vi "View.vi"(8 "error out":errorcluster, 11 "2-Axis Stage":refnum<class "2-Axis Stage Async API.lvclass">) -> (0 "error out":errorcluster)   [LabVIEW 2022 SP3, in "Control.lvlib"]
uses:
  Control.lvlib
  Interfaces/2-Axis Stage API/2-Axis Stage Async API.lvclass
panel:
  out "XY Position Graph":cluster{"X":dbl, "Y":dbl}[](graph)
  in  "Abort Motion":bool
  in  "Home Stage":bool
  in  "Move Stage":bool
  in  "Y-Destination":dbl
  in  "X-Destination":dbl
  in  "Clear Error":bool
  out "Y-Speed":dbl
  in  "Set Y-Speed":u16
  in  "Set Y-Acceleration":u16
  out "Y-Current Speed":dbl
  out "Y-Acceleration":dbl
  out "Y-Homed":bool
  out "Y-Moving":bool
  out "Y-Position":dbl
  out "X-Speed":dbl
  in  "Set X-Speed":u16
  in  "Set X-Acceleration":u16
  out "X-Current Speed":dbl
  out "X-Acceleration":dbl
  out "X-Homed":bool
  out "X-Moving":bool
  out "X-Position":dbl
  out "Stage Error":errorcluster
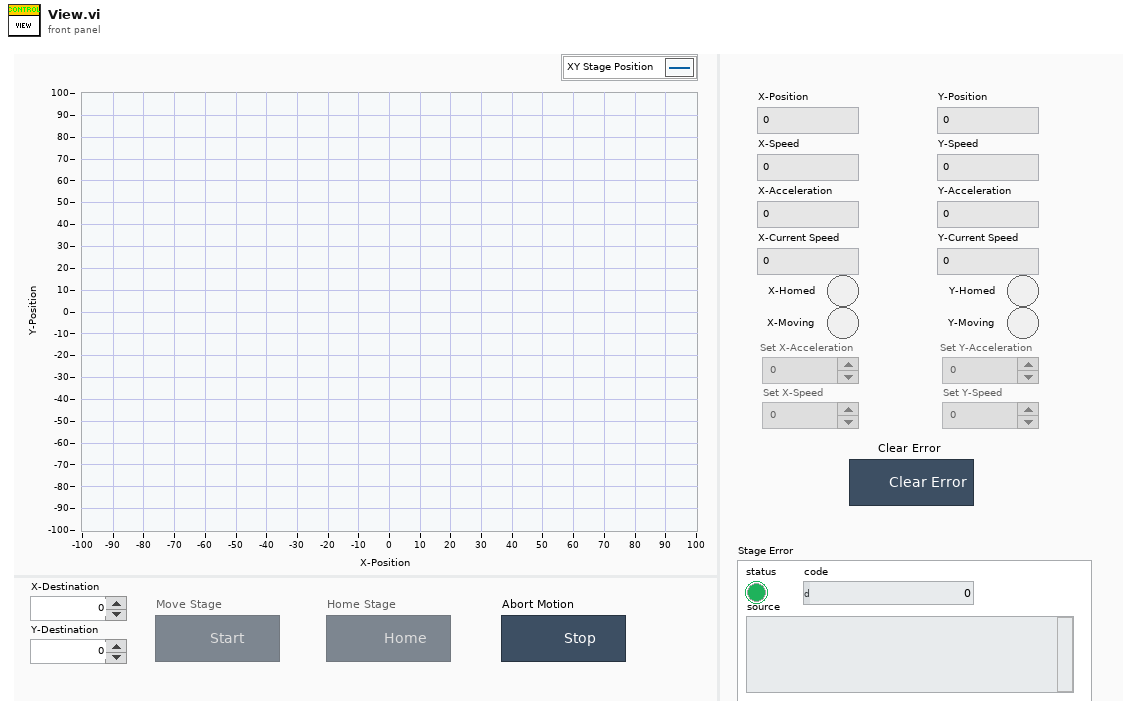
[diagram p1: front panel]
types:
  T1 = enum32{"Invalid", "Standard", "Closed", "Hidden", "Minimized", "Maximized"}
  T2 = enum32{"invalid app kind", "Development System", "Run Time System", "Student Edition", "Embedded LabVIEW", "Evaluation", "Custom"}
  T3 = enum8{"Enabled", "Disabled", "Disabled and Grayed Out"}
  T4 = cluster{"Current Position X":dbl, "Current Position Y":dbl}[]
  T5 = cluster{"Core":cluster{"Current VI Reference":refnum<vi>, "Close Panel on Exit?":bool}, "2-Axis Stage":refnum<class "2-Axis Stage Async API.lvclass">}
  T6 = cluster{"Current VI Reference":refnum<vi>, "Close Panel on Exit?":bool}
  T7 = cluster{"Event Registration Refnum":refnum<event-registration>, "Event Registration Refnum":refnum<event-registration>}
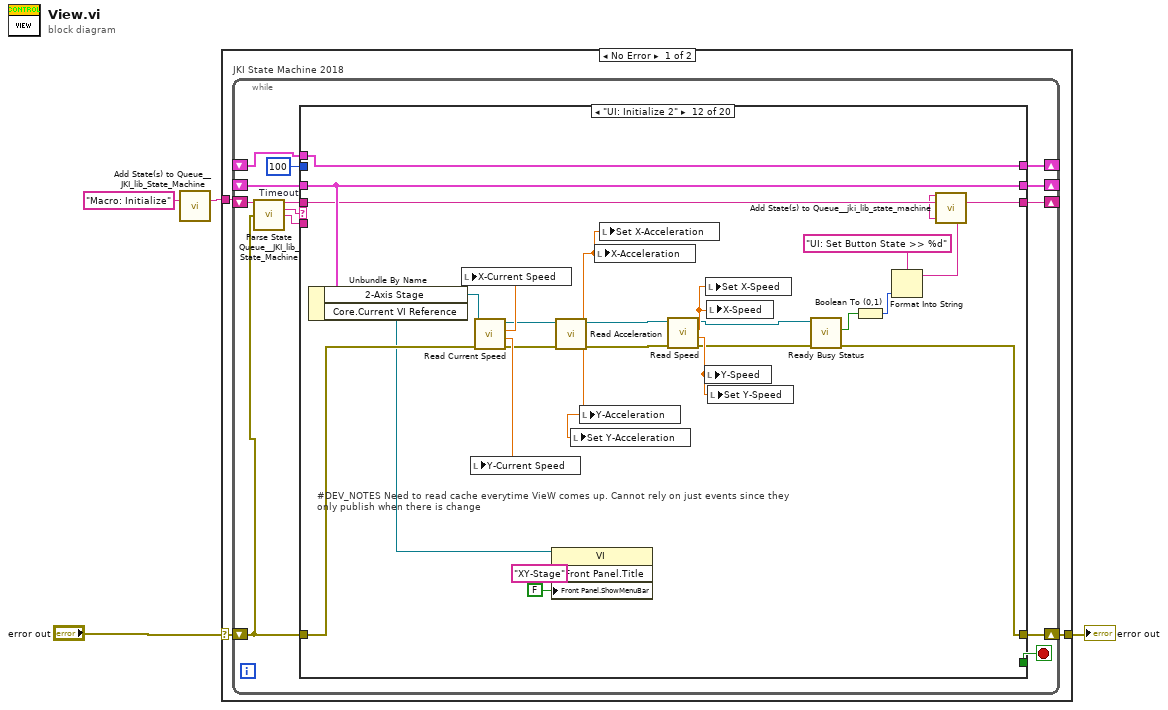
[diagram p0: block diagram]
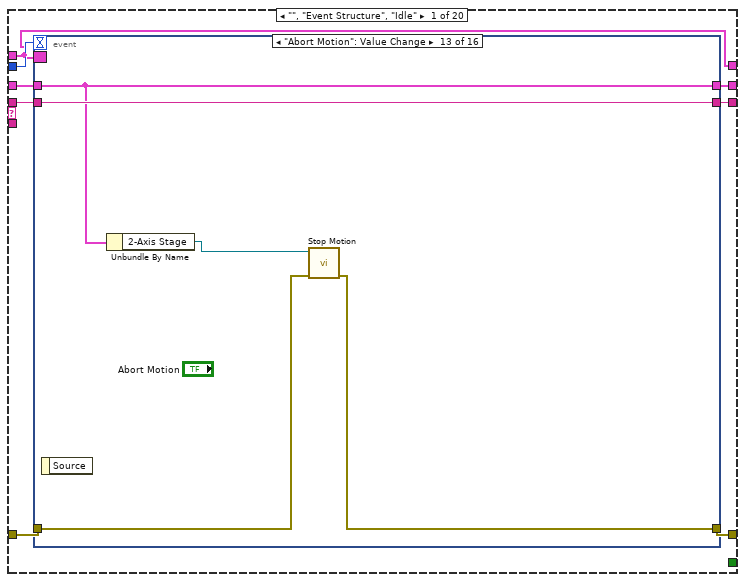
[diagram p2: hidden frame]
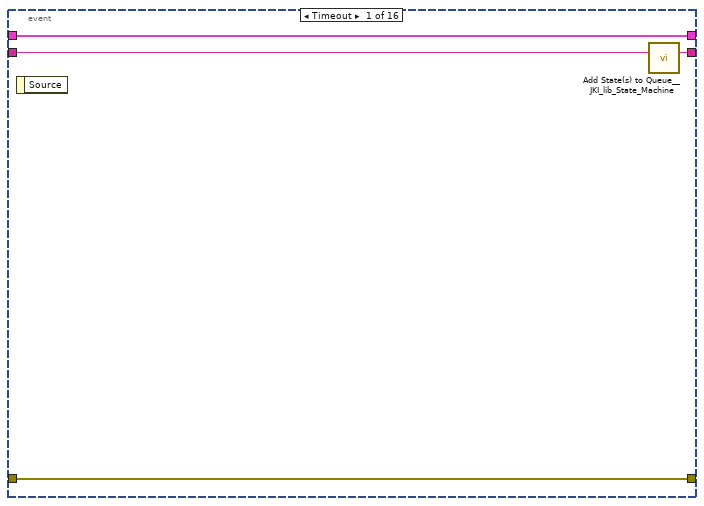
[diagram p3: hidden frame]
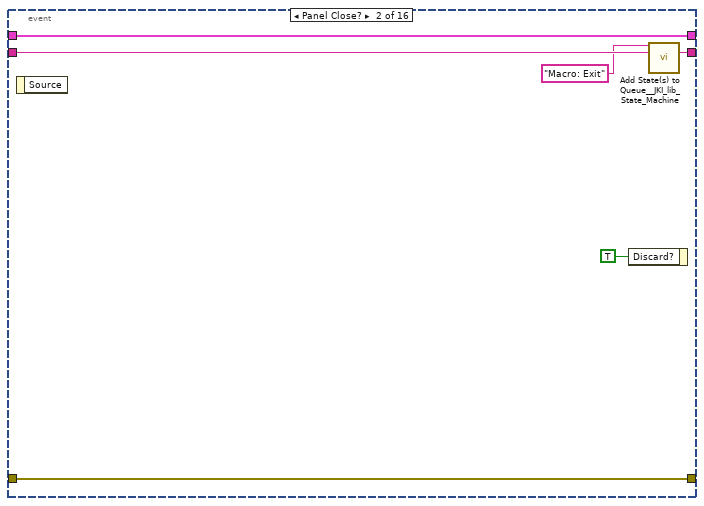
[diagram p4: hidden frame]
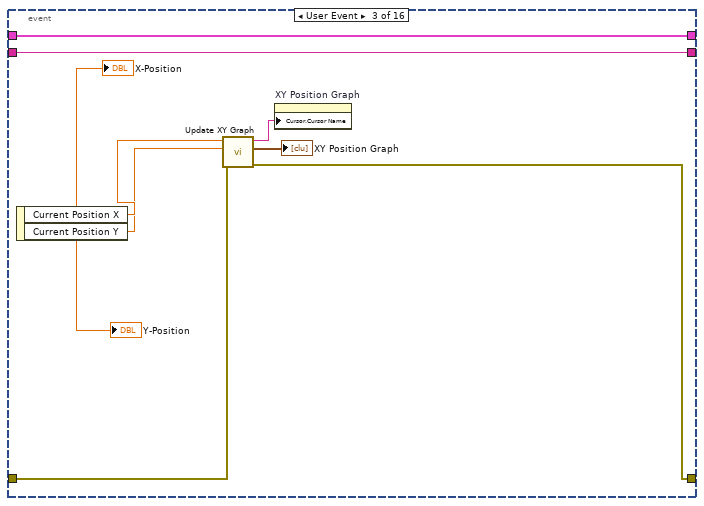
[diagram p5: hidden frame]
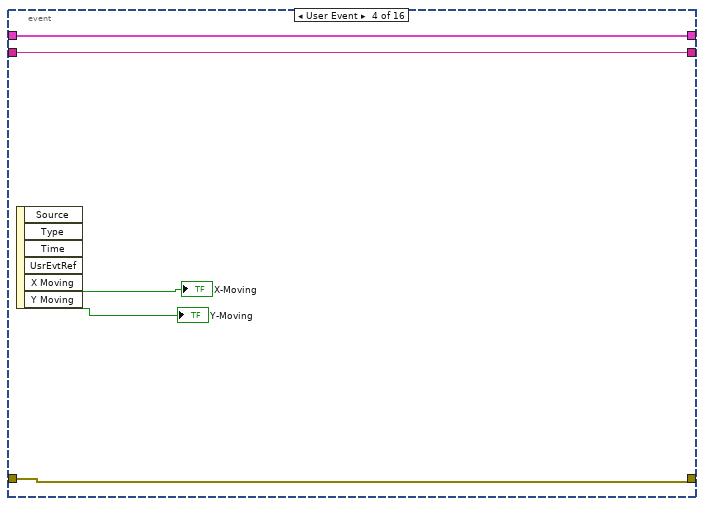
[diagram p6: hidden frame]
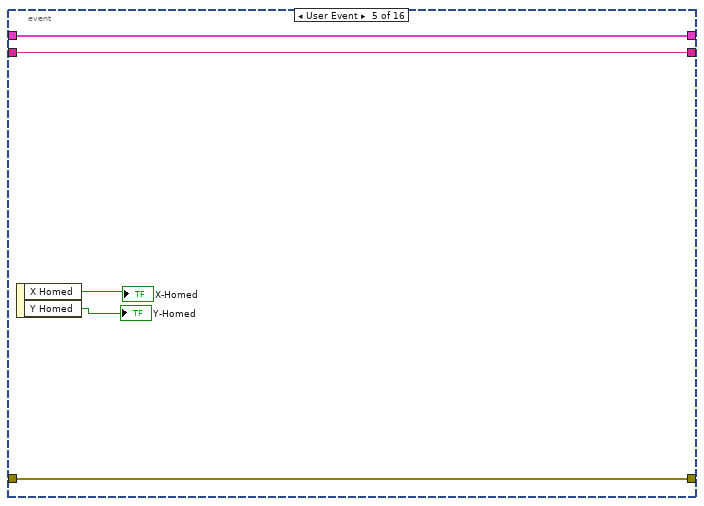
[diagram p7: hidden frame]
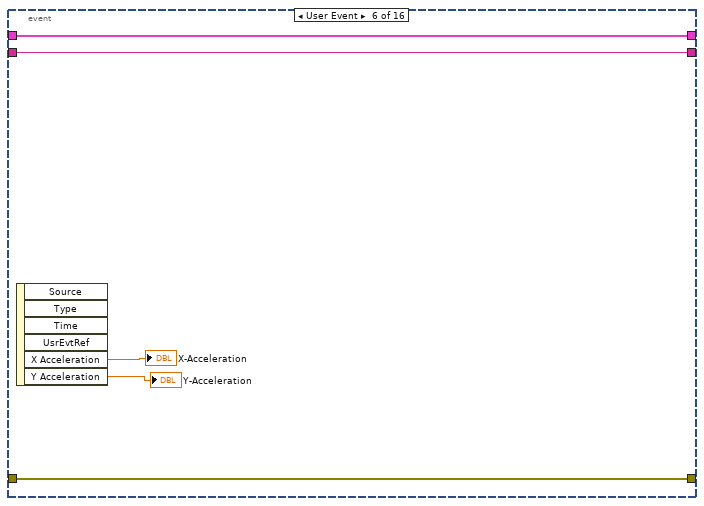
[diagram p8: hidden frame]
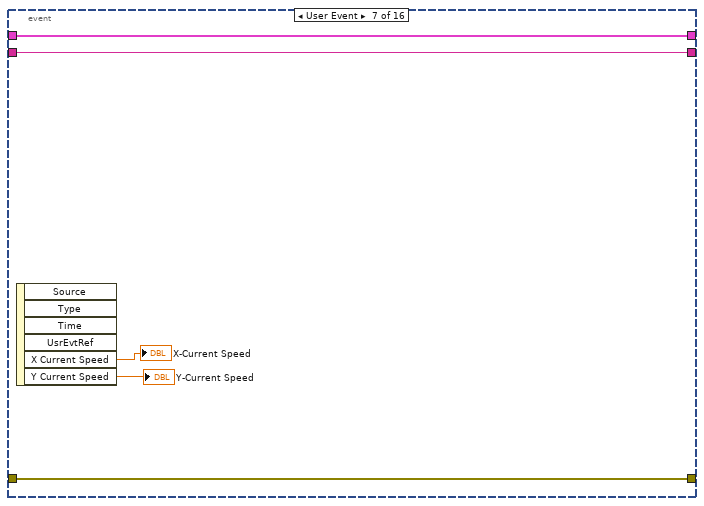
[diagram p9: hidden frame]
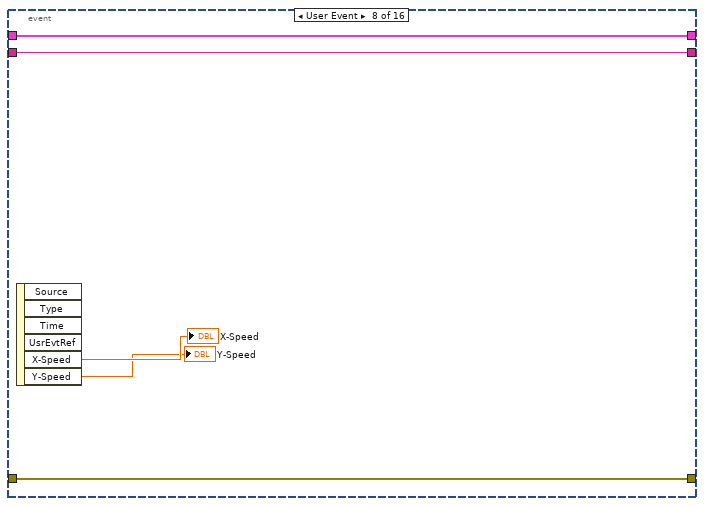
[diagram p10: hidden frame]
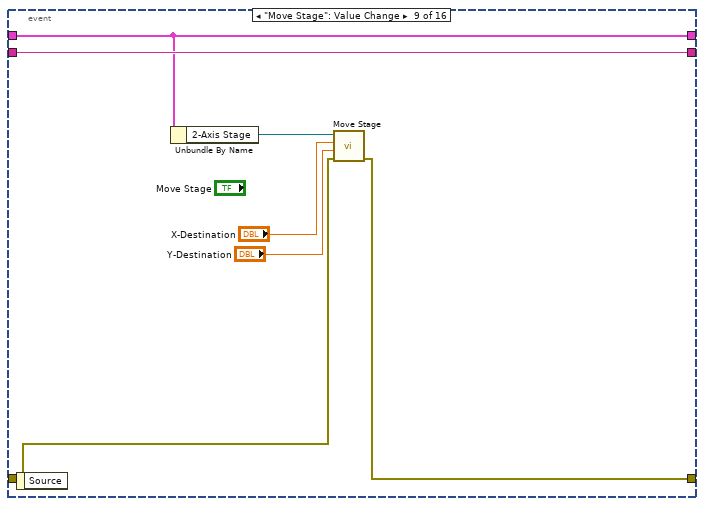
[diagram p11: hidden frame]
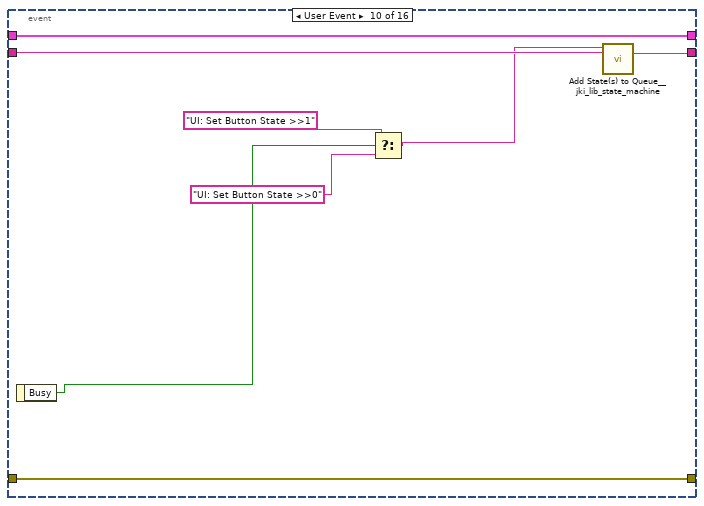
[diagram p12: hidden frame]
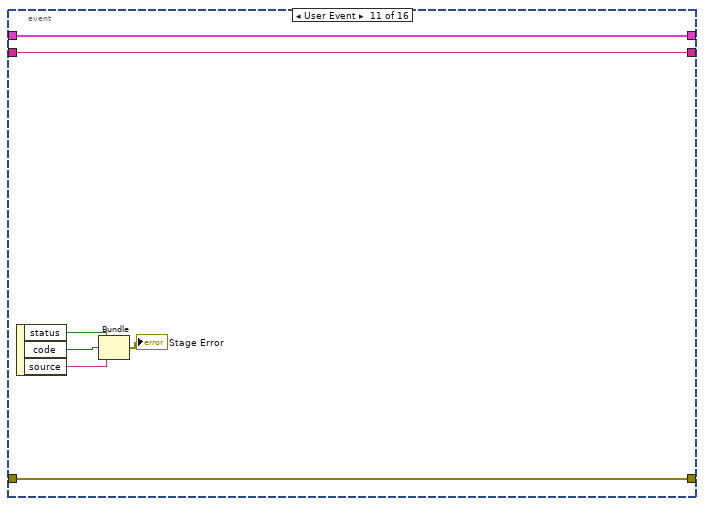
[diagram p13: hidden frame]
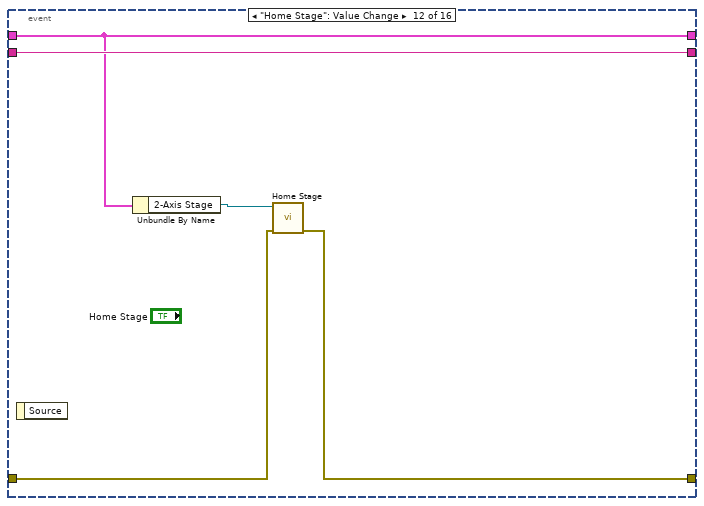
[diagram p14: hidden frame]
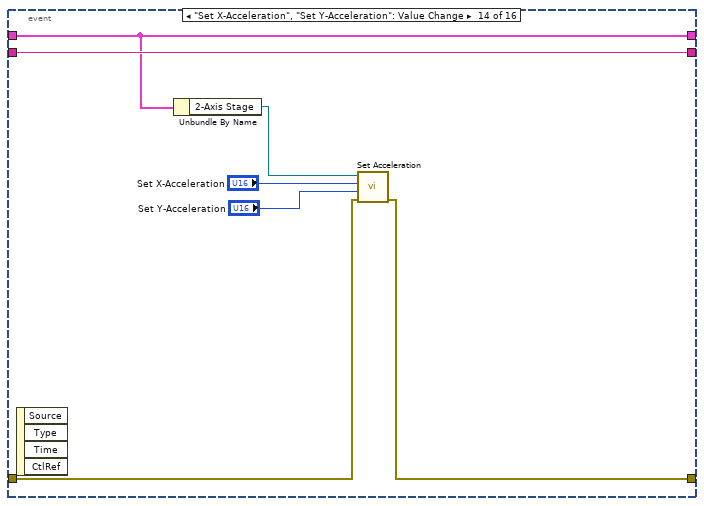
[diagram p15: hidden frame]
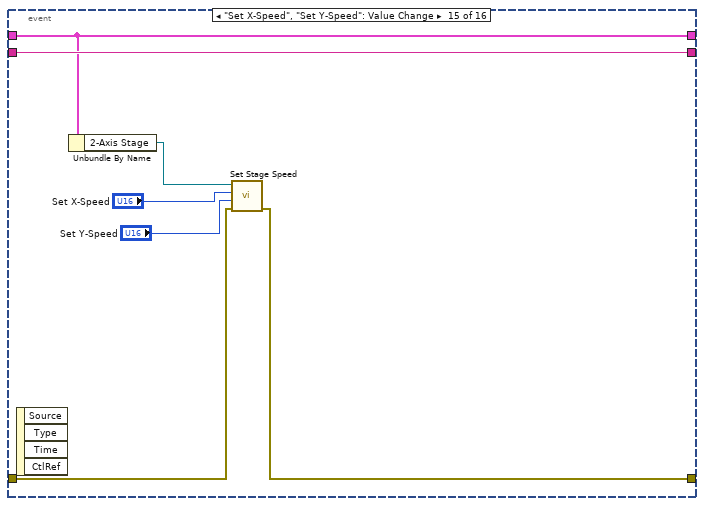
[diagram p16: hidden frame]
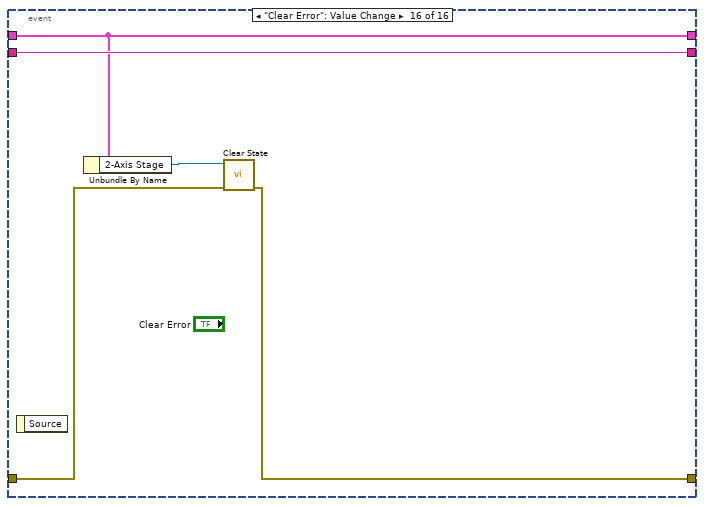
[diagram p17: hidden frame]
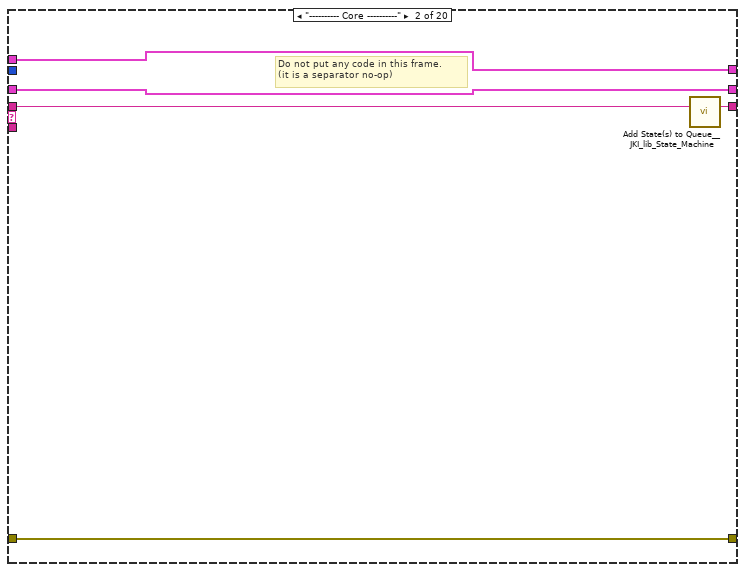
[diagram p18: hidden frame]
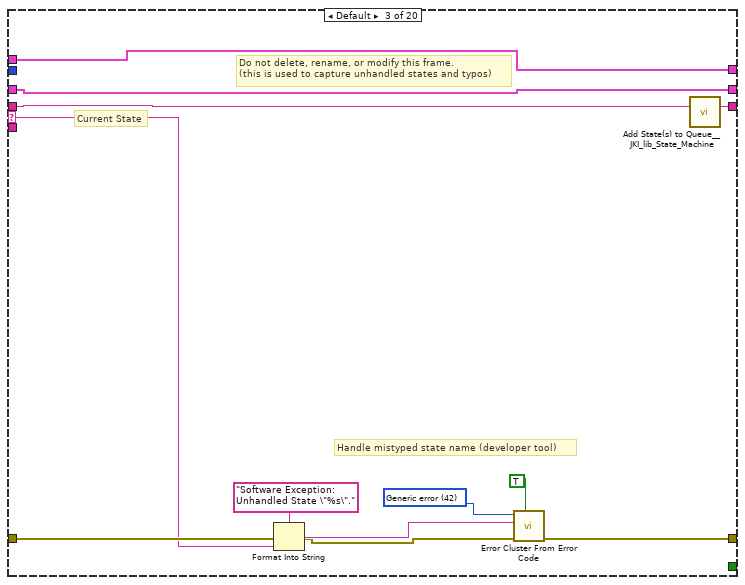
[diagram p19: hidden frame]
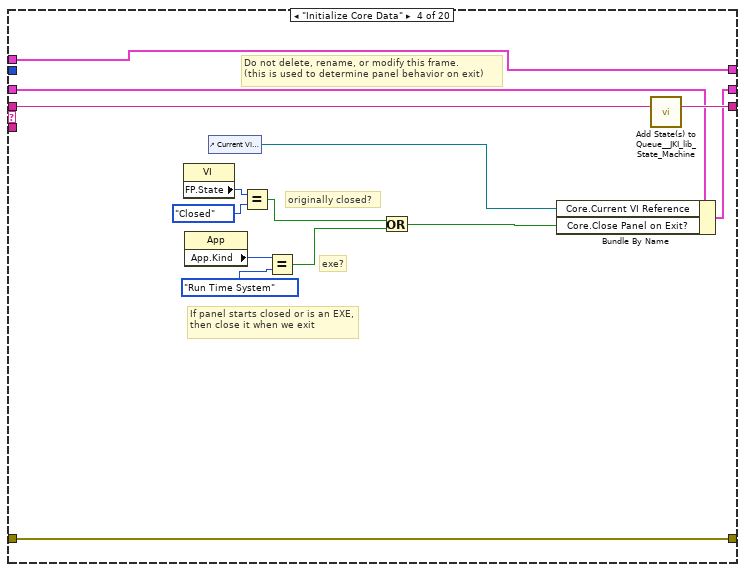
[diagram p20: hidden frame]
diagram:
  n1 = call <vilib>:"Add State(s) to Queue__JKI_lib_State_Machine.vi"("State(s) in (\"\")"="Macro: Initialize") -> ("States Out"=w1:string)  [unwired: 14 in]
  n2 = case shown="No Error" "error out" {
    selector: "error out" -> [w7 _]
    tunnel: [w6 _] -> w3
    tunnel: w1 -> [w5 _]
    frame No Error {
      n3 = while "JKI State Machine 2018" {
        shift-right: [w13] -> _
        shift-left: _ -> [w12]
        shift-right: [w16] -> w6
        shift-left: w7 -> [w10]
        shift-right: [w15] -> _
        shift-left: w5 -> [w17]
        shift-right: [w9] -> _
        shift-left: _ -> [w8]
        stop <- w14 stop-if-true
        w11 = 100  # Timeout
        n4 = call <vilib>:"Parse State Queue__JKI_lib_State_Machine.vi"("State Queue"=w17, "Error In (no error)"=w10) -> ("Remaining States"=w19:string, "Current State"=w20:string, "Arguments"=w18:string)  [unwired: 11 in]
        n5 = case shown="\"UI: Initialize 2\"" w20 {
          selector: w20 -> [_ _ w129 _ _ _ _ _ _ _ _ _ _ _ _ _ _ _ _ _]
          tunnel: w19 -> [w28 w127 w133 w153 w160 w166 w171 w178 w185 w190 w213 w224 w256 w278 w290 w360 w366 w377 w382 w388]
          tunnel: w18 -> [_ _ _ _ _ _ _ _ _ _ _ _ w245 w273 w284 _ _ _ _ _]
          tunnel: w12 -> [w26 w124 w131 w146 w157 w164 w168 _ w180 w187 w210 w228 w247 w276 w286 w357 w363 w374 w379 w387]
          tunnel: [w25 w125 w135 w150 errorcluster {"status"=FALSE, "code"=0, "source"=""} ("error out") w163 w169 w175 w181 w188 w195 w219 w242 w274 w287 w358 w364 w375 w380 w383] -> w16
          tunnel: w10 -> [w24 w125 w134 w150 w154 w163 w169 w175 w182 w188 w202 w226 w241 w275 w288 w358 w364 w375 w380 w384]
          tunnel: [w27 w126 w132 w152 w159 w165 w170 w177 w184 w189 w212 w225 w256 w277 w289 w359 w365 w376 w381 w388] -> w15
          tunnel: [_ _ _ _ _ TRUE _ _ _ _ _ _ _ _ _ _ _ _ _ _] -> w14
          tunnel: [w23 w124 w131 w151 w157 w164 w168 w176 w180 w187 w210 w228 w247 w276 w286 w357 w363 w374 w379 w387] -> w13
          tunnel: w11 -> [w22 _ _ _ _ _ _ _ _ _ _ _ _ _ _ _ _ _ _ _]
          tunnel: [w21 w123 w128 w140 w155 w161 w167 w172 w179 w186 w211 w239 w248 w272 w283 w356 w362 w367 w378 w385] -> w9
          tunnel: w8 -> [w21 w123 w128 w140 w155 w161 w167 w172 w179 w186 w211 w239 w248 w272 w283 w356 w362 w367 w378 _]
          frame "", "Event Structure", "Idle" {
            n6 = event shown="[12] \"Abort Motion\": Value Change" {
              selector: w21 -> [_ _ _ _ _ _ _ _ _ _ _ _ _ _ _ _]
              dyn-events: _ -> [_ _ _ _ _ _ _ _ _ _ _ _ _ _ _ _]
              timeout: w22 -> [_ _ _ _ _ _ _ _ _ _ _ _ _ _ _ _]
              tunnel: w28 -> [w32 w38 w45 w51 w56 w61 w66 w71 w78 w83 w93 w98 w103 w110 w117 w122]
              tunnel: [w31 w37 w45 w51 w56 w61 w66 w71 w78 w84 w93 w98 w103 w110 w117 w122] -> w27
              tunnel: w26 -> [w29 w35 w46 w50 w55 w60 w65 w70 w77 w86 w92 w97 w102 w109 w116 w121]
              tunnel: [w30 w36 w39 w47 w52 w57 w62 w67 w72 w85 w87 w94 w100 w104 w113 w118] -> w25
              tunnel: w24 -> [w30 w36 w40 w47 w52 w57 w62 w67 w73 w85 w87 w95 w99 w105 w114 w119]
              tunnel: [w29 w35 w46 w50 w55 w60 w65 w70 w77 w86 w92 w97 w102 w109 w116 w121] -> w23
              event Timeout {
                n7 = event-data() -> ()  [unwired: 1 in, 1 out]
                n8 = call <vilib>:"Add State(s) to Queue__JKI_lib_State_Machine.vi"("State(s) in (\"\")"=w32) -> ("States Out"=w31:string)  [unwired: 14 in]
              }
              event Panel Close? {
                n9 = event-data() -> ()  [unwired: 1 in, 1 out]
                n10 = event-data("Discard?"=TRUE) -> ()  [unwired: 1 in, 1 out]
                n11 = call <vilib>:"Add State(s) to Queue__JKI_lib_State_Machine.vi"("State(s) in Front (\"\")"="Macro: Exit", "State(s) in (\"\")"=w38) -> ("States Out"=w37:string)  [unwired: 13 in]
              }
              event User Event {
                n12 = event-data() -> ("Current Position X"=w43:dbl, "Current Position Y"=w42:dbl)  [unwired: 1 in]
                "Y-Position" <- w42
                "X-Position" <- w43
                n13 = call "Update XY Graph.vi"("error in (no error)"=w40, "Current Position Y"=w42, "Current Position X"=w43) -> ("error out"=w39:errorcluster, "Array"=→"XY Position Graph":T4, "String"=w41:string)  [unwired: 6 in]
                n14 = property on="XY Position Graph" class="XYGraph (strict)"("Cursor.Cursor Name"=w41) -> ()  [unwired: 2 in, 2 out]
              }
              event User Event {
                n15 = event-data() -> ("X Moving"=→"X-Moving":bool, "Y Moving"=→"Y-Moving":bool)  [unwired: 1 in, 4 out]
              }
              event User Event {
                n16 = event-data() -> ("X Homed"=→"X-Homed":bool, "Y Homed"=→"Y-Homed":bool)  [unwired: 1 in]
              }
              event User Event {
                n17 = event-data() -> ("X Acceleration"=→"X-Acceleration":dbl, "Y Acceleration"=→"Y-Acceleration":dbl)  [unwired: 1 in, 4 out]
              }
              event User Event {
                n18 = event-data() -> ("X Current Speed"=→"X-Current Speed":dbl, "Y Current Speed"=→"Y-Current Speed":dbl)  [unwired: 1 in, 4 out]
              }
              event User Event {
                n19 = event-data() -> ("X-Speed"=→"X-Speed":dbl, "Y-Speed"=→"Y-Speed":dbl)  [unwired: 1 in, 4 out]
              }
              event "Move Stage": Value Change {
                n20 = event-data() -> ()  [unwired: 1 in, 1 out]
                n21 = Unbundle By Name(w77) -> ("2-Axis Stage"=w76:refnum<class "2-Axis Stage Async API.lvclass">)
                n22 = call-dynamic "Move Stage.vi"("error in (no error)"=w73, "Y Axis"="Y-Destination", "X Axis"="X-Destination", "2-Axis Stage in"=w76) -> ("error out"=w72:errorcluster)  [unwired: 6 in, 1 out]
              }
              event User Event {
                n23 = event-data() -> ("Busy"=w82:bool)  [unwired: 1 in]
                n24 = Select(t="UI: Set Button State >>1", s=w82, f="UI: Set Button State >>0") -> (s? t:f=w79:string)
                n25 = call <vilib>:"Add State(s) to Queue__jki_lib_state_machine.vi"("State(s) in Front (\"\")"=w79, "State(s) in (\"\")"=w83) -> ("States Out"=w84:string)  [unwired: 13 in]
              }
              event User Event {
                n26 = event-data() -> ("status"=w91:bool, "code"=w90:i32, "source"=w89:string)  [unwired: 1 in]
                n27 = Bundle("status"=w91, "code"=w90, "source"=w89) -> (→"Stage Error":errorcluster)  [unwired: 1 in]
              }
              event "Home Stage": Value Change {
                n28 = event-data() -> ()  [unwired: 1 in, 1 out]
                n29 = Unbundle By Name(w97) -> ("2-Axis Stage"=w96:refnum<class "2-Axis Stage Async API.lvclass">)
                n30 = call-dynamic "Home Stage.vi"("error in (no error)"=w95, "2-Axis Async Home in"=w96) -> ("error out"=w94:errorcluster)  [unwired: 8 in, 1 out]
              }
              event "Abort Motion": Value Change {
                n31 = event-data() -> ()  [unwired: 1 in, 1 out]
                n32 = Unbundle By Name(w102) -> ("2-Axis Stage"=w101:refnum<class "2-Axis Stage Async API.lvclass">)
                n33 = call-dynamic "Stop Motion.vi"("error in (no error)"=w99, "2-Axis Stage in"=w101) -> ("error out"=w100:errorcluster)  [unwired: 8 in, 1 out]
              }
              event "Set X-Acceleration", "Set Y-Acceleration": Value Change {
                n34 = event-data() -> ()  [unwired: 1 in, 4 out]
                n35 = Unbundle By Name(w109) -> ("2-Axis Stage"=w108:refnum<class "2-Axis Stage Async API.lvclass">)
                n36 = call-dynamic "Set Acceleration.vi"("error in (no error)"=w105, "Y Axis"="Set Y-Acceleration", "X Axis"="Set X-Acceleration", "2-Axis Stage in"=w108) -> ("error out"=w104:errorcluster)  [unwired: 6 in, 1 out]
              }
              event "Set X-Speed", "Set Y-Speed": Value Change {
                n37 = event-data() -> ()  [unwired: 1 in, 4 out]
                n38 = Unbundle By Name(w116) -> ("2-Axis Stage"=w115:refnum<class "2-Axis Stage Async API.lvclass">)
                n39 = call-dynamic "Set Stage Speed.vi"("error in (no error)"=w114, "Y Axis"="Set Y-Speed", "X Axis"="Set X-Speed", "2-Axis Stage in"=w115) -> ("error out"=w113:errorcluster)  [unwired: 6 in, 1 out]
              }
              event "Clear Error": Value Change {
                n40 = event-data() -> ()  [unwired: 1 in, 1 out]
                n41 = Unbundle By Name(w121) -> ("2-Axis Stage"=w120:refnum<class "2-Axis Stage Async API.lvclass">)
                n42 = call-dynamic "Clear State.vi"("error in (no error)"=w119, "2-Axis Stage Status in"=w120) -> ("error out"=w118:errorcluster)  [unwired: 8 in, 1 out]
              }
            }
          }
          frame "---------- Core ----------" {
            # "Do not put any code in this frame.\n(it is a separator no-op)"
            n43 = call <vilib>:"Add State(s) to Queue__JKI_lib_State_Machine.vi"("State(s) in (\"\")"=w127) -> ("States Out"=w126:string)  [unwired: 14 in]
          }
          frame Default {
            w138 = 42 items=["No error", "Argument error", "Memory is full", "Out of zone", "End of file", "File already open", "Generic file I/O error", "File not found", "File permission error", "Disk is full", "Duplicate path", "Too many files open", "System feature not enabled", "Resource file not found", "Cannot add resource", "Resource not found", "Image not found", "Image memory error", "Pen does not exist", "Config type invalid", "Config token not found", "Config parse error", "Config memory error", "Bad external code format", "Bad external code offset", "External code not present", "Null window", "Destroy window error", "Null menu", "Print aborted", "Bad print record", "Print driver error", "Windows error during printing", "Memory error during printing", "Print dialog error", "Generic print error", "Invalid device refnum", "Device not found", "Device parameter error", "Device unit error", "Cannot open device", "Device call aborted", "Generic error", "Cancelled by user", "Object ID too low", "Object ID too high", "Object not in heap", "Unknown heap", "Unknown object (invalid DefProc)", "Unknown object (DefProc not in table)", "Message out of range", "Invalid (null) method", "Unknown message", "Manager call not supported", "Bad address", "Network operation in progress", "Network operation timed out", "Connection is busy", "Network attribute not supported", "Network error", "Address in use", "System out of memory", "Connection aborted", "Connection refused", "Not connected", "Already connected", "Connection closed", "Initialization error (interapplication manager)", "Bad occurrence", "Wait on unbound occurrence handler", "Occurrence queue overflow", "Datalog type conflict", "Unused", "Unrecognized type (interapplication manager)", "Memory corrupt", "Failed to make temporary DLL", "Old CIN version", "Drag socket not found", "Failed to load drop-object", "Failed to register OLE object", "Failed to release OLE object", "Format specifier type mismatch", "Unknown format specifier", "Too few format specifiers", "Too many format specifiers", "Scan failed", "Newer CIN version", "Error converting to variant", "Runtime menu error", "Password tampered", "Variant attribute not found", "Incompatible variant data type", "Event data is not available", "Event Store is not present", "Occurrence is not found", "Event Queue is not created", "Event info is not available", "Refnum passed is NULL", "Error retrieving Class GUID", "Error retrieving CoClass GUID", "Error retrieving TypeLib GUID.", "Bad built application magic bytes.", "Specific driver is different from the specific driver associated with the Logical Name.", "There is no session opened to the class driver.", "Max Error", "MAX - Error with config objects", "MAX - Error loading configuration", "MAX - Group not supported"]
            # "Current State"
            # "Do not delete, rename, or modify this frame.\n(this is used to capture unhandled states and typos)"
            # "Handle mistyped state name (developer tool)"
            n44 = Format Into String(format string="Software Exception: Unhandled State \"%s\"." ("message"), error in=w134, w129) -> (resulting string=w137:string, error out=w136:errorcluster)  [unwired: 1 in]
            n45 = call <vilib>:"Error Cluster From Error Code.vi"("show call chain? (False)"=TRUE, "error in (no error)"=w136, "error message (\"\")"=w137, "error code (0)"=w138) -> ("error out"=w135:errorcluster)  [unwired: 5 in]
            n46 = call <vilib>:"Add State(s) to Queue__JKI_lib_State_Machine.vi"("State(s) in (\"\")"=w133) -> ("States Out"=w132:string)  [unwired: 14 in]
          }
          frame "Initialize Core Data" {
            # "Do not delete, rename, or modify this frame.\n(this is used to determine panel behavior on exit)"
            # "originally closed?"
            # "exe?"
            # "If panel starts closed or is an EXE, then close it when we exit"
            n47 = property class="VI"() -> ("FP.State"=w143:T1)  [unwired: 2 in, 2 out]
            n48 = property class="App"() -> ("App.Kind"=w149:T2)  [unwired: 2 in, 2 out]
            n49 = control-ref of="Current VI Reference"() -> (w144:refnum<vi>)
            n50 = Equal?(x=w143, y=T1."Closed" ("Front Panel Window:State")) -> (x = y?=w141:bool)
            n51 = Equal?(x=w149, y=T2."Run Time System" ("Application:Kind")) -> (x = y?=w147:bool)
            n52 = Or(x=w141, y=w147) -> (x .or. y?=w145:bool)
            n53 = Bundle By Name(cluster=w146, "Core.Current VI Reference"=w144, "Core.Close Panel on Exit?"=w145) -> (w151:T5)
            n54 = call <vilib>:"Add State(s) to Queue__JKI_lib_State_Machine.vi"("State(s) in (\"\")"=w153) -> ("States Out"=w152:string)  [unwired: 14 in]
          }
          frame "Error Handler" {
            # "Handle any errors here.\nYou can also output any states to clean-up after errors occur"
            # "Clear error"
            n55 = local write "Stage Error"(w154) -> ()
            n56 = call <vilib>:"Add State(s) to Queue__JKI_lib_State_Machine.vi"("State(s) in Front (\"\")"="/* Post Error States", "State(s) in (\"\")"=w160) -> ("States Out"=w159:string)  [unwired: 13 in]
          }
          frame "Exit" {
            # "Do not put any code in this frame.\n(No errors that occur here will be handled.)"
            n57 = call <vilib>:"Add State(s) to Queue__JKI_lib_State_Machine.vi"("State(s) in (\"\")"=w166) -> ("States Out"=w165:string)  [unwired: 14 in]
          }
          frame "---------- Data ----------" {
            # "Do not put any code in this frame.\n(It is a separator no-op. You can make a copy of this frame to create a new Data frame)"
            n58 = call <vilib>:"Add State(s) to Queue__JKI_lib_State_Machine.vi"("State(s) in (\"\")"=w171) -> ("States Out"=w170:string)  [unwired: 14 in]
          }
          frame "Data: Initialize" {
            w174 = T6 {"Current VI Reference"=refnum, "Close Panel on Exit?"=FALSE}  # Core
            # "Data names and types of shift register data are defined by this bundle."
            # "Initialize the shift-register data, here.\n(data names are defined by what you wire into the bundle function)"
            n59 = Bundle("Core"=w174, "2-Axis Stage"="2-Axis Stage") -> (w176:T5)  [unwired: 1 in]
            n60 = call <vilib>:"Add State(s) to Queue__JKI_lib_State_Machine.vi"("State(s) in (\"\")"=w178) -> ("States Out"=w177:string)  [unwired: 14 in]
          }
          frame "Data: Cleanup" {
            # "Cleanup any data and references, here.\n(this is called automatically, by the Macro: Exit)"
            n61 = Unbundle By Name(w180) -> ("Core.Current VI Reference"=w183:refnum<vi>)
            n62 = Close Reference(reference=w183, error in (no error)=w182) -> (error out=w181:errorcluster)
            n63 = call <vilib>:"Add State(s) to Queue__JKI_lib_State_Machine.vi"("State(s) in (\"\")"=w185) -> ("States Out"=w184:string)  [unwired: 14 in]
          }
          frame "---------- UI ----------" {
            # "Do not put any code in this frame.\n(It is a separator no-op. You can make a copy of this frame to create a new UI frame)"
            n64 = call <vilib>:"Add State(s) to Queue__JKI_lib_State_Machine.vi"("State(s) in (\"\")"=w190) -> ("States Out"=w189:string)  [unwired: 14 in]
          }
          frame "UI: Initialize 1" {
            # "Initialize the User Interface, here.\n(this is called automatically, by the Macro: Init)"
            n65 = Unbundle By Name(w210) -> ("2-Axis Stage"=w207:refnum<class "2-Axis Stage Async API.lvclass">)
            n66 = call-dynamic "Read Current Position.vi"("error in (no error)"=w202, "2-Axis Stage Status in"=w207) -> ("error out"=w204:errorcluster, "Y Position"=w193:dbl, "X Position"=w194:dbl, "2-Axis Stage Status out"=w206:refnum<class "2-Axis Stage Async API.lvclass">)  [unwired: 6 in]
            n67 = call "Update XY Graph.vi"("Current Position Y"=w193, "Current Position X"=w194) -> ("Array"=w192:T4, "String"=w191:string)  [unwired: 7 in, 1 out]
            n68 = local write "X-Position"(w194) -> ()
            n69 = local write "Y-Position"(w193) -> ()
            n70 = local write "XY Position Graph"(w192) -> ()
            n71 = property on="XY Position Graph" class="XYGraph (strict)"("Cursor.Cursor Name"=w191) -> ()  [unwired: 2 in, 2 out]
            n72 = call-dynamic "Read Moving Flags.vi"("error in (no error)"=w204, "2-Axis Stage Status in"=w206) -> ("error out"=w203:errorcluster, "Y-Axis Moving"=w208:bool, "X-Axis Moving"=w209:bool, "2-Axis Stage Status out"=w205:refnum<class "2-Axis Stage Async API.lvclass">)  [unwired: 6 in]
            n73 = local write "Y-Moving"(w208) -> ()
            n74 = local write "X-Moving"(w209) -> ()
            n75 = call-dynamic "Read Stage Homed.vi"("error in (no error)"=w203, "2-Axis Stage Status in"=w205) -> ("error out"=w195:errorcluster, "Y-Axis Homed Moving"=w200:bool, "X-Axis Homed"=w201:bool)  [unwired: 6 in, 1 out]
            n76 = local write "Y-Homed"(w200) -> ()
            n77 = And(x=w201, y=w200) -> (x .and. y?=w199:bool)
            n78 = Select(t=T3."Enabled" ("Disabled"), s=w199, f=T3."Disabled and Grayed Out" ("Disabled")) -> (s? t:f=w197:T3)
            n79 = local write "X-Homed"(w201) -> ()
            n80 = property on="Move Stage" class="Bool"("DisabledEnum"=w197) -> ()  [unwired: 2 in, 2 out]
            n81 = call <vilib>:"Add State(s) to Queue__JKI_lib_State_Machine.vi"("State(s) in (\"\")"=w213) -> ("States Out"=w212:string)  [unwired: 14 in]
          }
          frame "UI: Initialize 2" {
            # "#DEV_NOTES Need to read cache everytime VieW comes up. Cannot rely on just events since they only publish when there is change"
            n82 = Unbundle By Name(w228) -> ("2-Axis Stage"=w227:refnum<class "2-Axis Stage Async API.lvclass">, "Core.Current VI Reference"=w216:refnum<vi>)
            n83 = call-dynamic "Read Current Speed.vi"("error in (no error)"=w226, "2-Axis Stage Status in"=w227) -> ("error out"=w235:errorcluster, "Y Current Speed"=w238:dbl, "X Current Speed"=w237:dbl, "2-Axis Stage Status out"=w236:refnum<class "2-Axis Stage Async API.lvclass">)  [unwired: 6 in]
            n84 = local write "X-Current Speed"(w237) -> ()
            n85 = local write "Y-Current Speed"(w238) -> ()
            n86 = property class="VI"(reference=w216, "Front Panel.Title"="XY-Stage" ("Front Panel Window:Title"), "Front Panel.ShowMenuBar"=FALSE ("Front Panel Window:Show Menu Bar")) -> ()  [unwired: 1 in, 2 out]
            n87 = call-dynamic "Read Acceleration.vi"("error in (no error)"=w235, "2-Axis Stage Status in"=w236) -> ("error out"=w233:errorcluster, "Y Acceleration"=w229:dbl, "X Acceleration"=w230:dbl, "2-Axis Stage Status out"=w234:refnum<class "2-Axis Stage Async API.lvclass">)  [unwired: 6 in]
            n88 = local write "Set Y-Acceleration"(w229) -> ()
            n89 = local write "Y-Acceleration"(w229) -> ()
            n90 = local write "X-Acceleration"(w230) -> ()
            n91 = local write "Set X-Acceleration"(w230) -> ()
            n92 = call-dynamic "Read Speed.vi"("error in (no error)"=w233, "2-Axis Stage Status in"=w234) -> ("error out"=w220:errorcluster, "Y-Axis Speed"=w231:dbl, "X-Axis Speed"=w232:dbl, "2-Axis Stage Status out"=w221:refnum<class "2-Axis Stage Async API.lvclass">)  [unwired: 6 in]
            n93 = local write "Y-Speed"(w231) -> ()
            n94 = local write "Set X-Speed"(w232) -> ()
            n95 = local write "X-Speed"(w232) -> ()
            n96 = local write "Set Y-Speed"(w231) -> ()
            n97 = call-dynamic "Ready Busy Status.vi"("error in (no error)"=w220, "2-Axis Stage Status in"=w221) -> ("error out"=w219:errorcluster, "Busy"=w218:bool)  [unwired: 7 in, 1 out]
            n98 = Boolean To (0,1)(Boolean=w218) -> (0, 1=w217:i16)
            n99 = Format Into String(format string="UI: Set Button State >> %d", w217) -> (resulting string=w222:string)  [unwired: 2 in, 1 out]
            n100 = call <vilib>:"Add State(s) to Queue__jki_lib_state_machine.vi"("State(s) in Front (\"\")"=w222, "State(s) in (\"\")"=w224) -> ("States Out"=w225:string)  [unwired: 13 in]
          }
          frame "UI: Set Button State" {
            n101 = Scan From String(format string="%d", input string=w245, error in=w241) -> (error out=w240:errorcluster, output 1=w243:i32)  [unwired: 2 in, 2 out]
            n102 = Unbundle By Name(w247) -> ("2-Axis Stage"=w246:refnum<class "2-Axis Stage Async API.lvclass">)
            n103 = case shown="1" w243 {
              tunnel: [T3."Enabled" ("Disabled") w270] -> w255
              tunnel: [T3."Disabled and Grayed Out" ("Disabled") T3."Enabled" ("Disabled")] -> w254
              tunnel: [w261 w270] -> w253
              tunnel: [w260 w269] -> w242
              tunnel: [w259 w270] -> w252
              tunnel: [w259 w270] -> w251
              tunnel: [w259 w270] -> w250
              tunnel: [w259 w270] -> w249
              tunnel: w246 -> [w258 _]
              tunnel: w240 -> [w257 w269]
              frame 0, Default {
                w259 = T3."Enabled" ("Disabled")
                n104 = call-dynamic "Read Stage Homed.vi"("error in (no error)"=w257, "2-Axis Stage Status in"=w258) -> ("error out"=w260:errorcluster, "Y-Axis Homed Moving"=w265:bool, "X-Axis Homed"=w266:bool)  [unwired: 6 in, 1 out]
                n105 = And(x=w266, y=w265) -> (x .and. y?=w264:bool)
                n106 = Select(t=T3."Enabled" ("Disabled"), s=w264, f=T3."Disabled and Grayed Out" ("Disabled")) -> (s? t:f=w261:T3)
              }
              frame 1 {
                w270 = T3."Disabled and Grayed Out" ("Disabled")
              }
            }
            n107 = property on="Abort Motion" class="Bool"("DisabledEnum"=w254) -> ()  [unwired: 2 in, 2 out]
            n108 = property on="Set Y-Speed" class="DigNum (strict)"("DisabledEnum"=w252) -> ()  [unwired: 2 in, 2 out]
            n109 = property on="Set X-Speed" class="DigNum (strict)"("DisabledEnum"=w251) -> ()  [unwired: 2 in, 2 out]
            n110 = property on="Set Y-Acceleration" class="DigNum (strict)"("DisabledEnum"=w250) -> ()  [unwired: 2 in, 2 out]
            n111 = property on="Set X-Acceleration" class="DigNum (strict)"("DisabledEnum"=w249) -> ()  [unwired: 2 in, 2 out]
            n112 = property on="Move Stage" class="Bool"("DisabledEnum"=w253) -> ()  [unwired: 2 in, 2 out]
            n113 = property on="Home Stage" class="Bool"("DisabledEnum"=w255) -> ()  [unwired: 2 in, 2 out]
          }
          frame "UI: Cursor Set" {
            # "Argument"
            # "Set and Unset Cursor Busy.\n(Usage: \"UI: Cursor Set >> Busy|Idle\")"
            n114 = case shown="\"Idle\", Default" w273 {
              tunnel: w275 -> [w280 w282]
              tunnel: [w279 w281] -> w274
              frame "Idle", Default {
                n115 = call <vilib>:"Unset Busy.vi"("error in (no error)"=w280) -> ("error out"=w279:errorcluster)  [unwired: 10 in]
              }
              frame "Busy" {
                n116 = call <vilib>:"Set Busy.vi"("error in (no error)"=w282) -> ("error out"=w281:errorcluster)  [unwired: 9 in, 1 out]
              }
            }
            n117 = call <vilib>:"Add State(s) to Queue__JKI_lib_State_Machine.vi"("State(s) in (\"\")"=w278) -> ("States Out"=w277:string)  [unwired: 14 in]
          }
          frame "UI: Front Panel State" {
            # "Argument"
            # "Set Front Panel Open or Closed\n(Usage: \"UI: Front Panel State >> Open|Close\")"
            n118 = Unbundle By Name(w286) -> ("Core.Current VI Reference"=w285:refnum<vi>)
            n119 = case shown="\"Minimize\", \"Minimized\"" w284 {
              tunnel: w288 -> [w296 w311 w322 w335 w348]
              tunnel: [w298 w312 w324 w337 w350] -> w287
              tunnel: w285 -> [w297 w309 w323 w336 w349]
              frame "Open", "Standard", Default {
                w291 = T1."Standard" ("State")
                n120 = property class="VI"(reference=w297, error in=w296) -> (reference out=w294:refnum<vi>, error out=w295:errorcluster, "FP.State"=w293:T1)
                n121 = Not Equal?(x=w293, y=w291) -> (x != y?=w292:bool)
                n122 = case shown="True" w292 {
                  tunnel: [w302 w304] -> w298
                  tunnel: w295 -> [w301 w304]
                  tunnel: w294 -> [w300 _]
                  tunnel: w291 -> [w299 _]
                  frame True {
                    n123 = invoke class="VI" method="FP.Open"(reference=w300, error in=w301, "Activate"=TRUE, "State"=w299) -> (error out=w302:errorcluster)  [unwired: 1 in, 4 out]
                  }
                  frame False {
                  }
                }
              }
              frame "Close", "Closed" {
                n124 = property class="VI"(reference=w309, error in=w311) -> (reference out=w308:refnum<vi>, error out=w310:errorcluster, "FP.State"=w306:T1)
                n125 = Not Equal?(x=w306, y=T1."Closed" ("Front Panel Window:State")) -> (x != y?=w305:bool)
                n126 = case shown="True" w305 {
                  tunnel: [w313 w316] -> w312
                  tunnel: w310 -> [w313 w315]
                  tunnel: w308 -> [_ w314]
                  frame False {
                  }
                  frame True {
                    n127 = invoke class="VI" method="FP.Close"(reference=w314, error in=w315) -> (error out=w316:errorcluster)  [unwired: 1 in, 2 out]
                  }
                }
              }
              frame "Hidden", "Hide" {
                w317 = T1."Hidden" ("State")
                n128 = property class="VI"(reference=w323, error in=w322) -> (reference out=w320:refnum<vi>, error out=w321:errorcluster, "FP.State"=w319:T1)
                n129 = Not Equal?(x=w319, y=w317) -> (x != y?=w318:bool)
                n130 = case shown="True" w318 {
                  tunnel: [w328 w329] -> w324
                  tunnel: w321 -> [w327 w329]
                  tunnel: w320 -> [w326 _]
                  tunnel: w317 -> [w325 _]
                  frame True {
                    n131 = invoke class="VI" method="FP.Open"(reference=w326, error in=w327, "State"=w325) -> (error out=w328:errorcluster)  [unwired: 2 in, 4 out]
                  }
                  frame False {
                  }
                }
              }
              frame "Minimize", "Minimized" {
                w330 = T1."Minimized" ("State")
                n132 = property class="VI"(reference=w336, error in=w335) -> (reference out=w333:refnum<vi>, error out=w334:errorcluster, "FP.State"=w332:T1)
                n133 = Not Equal?(x=w332, y=w330) -> (x != y?=w331:bool)
                n134 = case shown="True" w331 {
                  tunnel: [w341 w342] -> w337
                  tunnel: w334 -> [w340 w342]
                  tunnel: w333 -> [w339 _]
                  tunnel: w330 -> [w338 _]
                  frame True {
                    n135 = invoke class="VI" method="FP.Open"(reference=w339, error in=w340, "State"=w338) -> (error out=w341:errorcluster)  [unwired: 2 in, 4 out]
                  }
                  frame False {
                  }
                }
              }
              frame "Maximize", "Maximized" {
                w343 = T1."Maximized" ("State")
                n136 = property class="VI"(reference=w349, error in=w348) -> (reference out=w346:refnum<vi>, error out=w347:errorcluster, "FP.State"=w345:T1)
                n137 = Not Equal?(x=w345, y=w343) -> (x != y?=w344:bool)
                n138 = case shown="True" w344 {
                  tunnel: [w354 w355] -> w350
                  tunnel: w347 -> [w353 w355]
                  tunnel: w346 -> [w352 _]
                  tunnel: w343 -> [w351 _]
                  frame True {
                    n139 = invoke class="VI" method="FP.Open"(reference=w352, error in=w353, "State"=w351) -> (error out=w354:errorcluster)  [unwired: 2 in, 4 out]
                  }
                  frame False {
                  }
                }
              }
            }
            n140 = call <vilib>:"Add State(s) to Queue__JKI_lib_State_Machine.vi"("State(s) in (\"\")"=w290) -> ("States Out"=w289:string)  [unwired: 14 in]
          }
          frame "---------- Macro ----------" {
            # "Do not put any code in this frame.\n(It is a separator no-op. You can make a copy of this frame to create a new Macro frame)"
            n141 = call <vilib>:"Add State(s) to Queue__JKI_lib_State_Machine.vi"("State(s) in (\"\")"=w360) -> ("States Out"=w359:string)  [unwired: 14 in]
          }
          frame "Macro: Initialize" {
            w361 = "Data: Initialize\nInitialize Core Data\nEvents: Register for Events\nUI: Initialize 1\nUI: Initialize 2\nUI: Front Panel State >> Open"  # Data: Initialize Initialize Core Data Events: Register for Events UI: Initialize 1 UI: Initialize 2 UI: Front Panel State >> Open
            # "Initialization Macro\n(This is called once, when the VI starts)"
            n142 = call <vilib>:"Add State(s) to Queue__JKI_lib_State_Machine.vi"("State(s) in Front (\"\")"=w361, "State(s) in (\"\")"=w366) -> ("States Out"=w365:string)  [unwired: 13 in]
          }
          frame "Macro: Exit" {
            # "Exit Macro\n(This is called once, when the VI exits)"
            n143 = Unbundle By Name(w374) -> ("Core.Close Panel on Exit?"=w373:bool)
            n144 = Select(t="UI: Front Panel State >> Close", s=w373, f="") -> (s? t:f=w370:string)
            n145 = call <vilib>:"Add State(s) to Queue__JKI_lib_State_Machine.vi"("State(s) in (\"\")"=w370, "State(s) at Back (\"\")"="Data: Cleanup\nExit") -> ("States Out"=w368:string)  [unwired: 13 in]
            n146 = call <vilib>:"Add State(s) to Queue__JKI_lib_State_Machine.vi"("State(s) in Front (\"\")"=w368, "State(s) in (\"\")"=w377) -> ("States Out"=w376:string)  [unwired: 13 in]
          }
          frame "---------- Events ----------" {
            # "Template Separator\n(You can make a copy of, or modify, this frame)"
            n147 = call <vilib>:"Add State(s) to Queue__JKI_lib_State_Machine.vi"("State(s) in (\"\")"=w382) -> ("States Out"=w381:string)  [unwired: 14 in]
          }
          frame "Events: Register for Events" {
            n148 = Unbundle By Name(w387) -> ("2-Axis Stage"=w386:refnum<class "2-Axis Stage Async API.lvclass">)
            n149 = call-dynamic "Register for Events.vi"("error in (no error)"=w384, "Async Coms in"=w386) -> ("error out"=w383:errorcluster, "Event Refnums"=w385:T7)  [unwired: 7 in, 1 out]
          }
        }
      }
    }
    frame Error {
    }
  }
  "error out" <- w3
